vi "FetchVal34980a.vi"(0 "IP Address":string="localhost", 5 "TCP port":u16=5025 min=1025 step=1, 7 "Circuit ID":i32=1016 format="%_4g", 11 "error in (no error)":errorcluster) -> (4 "Value":dbl format="%#_10e", 15 "Error out":errorcluster)   [LabVIEW 2009]
doc: "Reads a value from the 34980. \nAssumes that you have scanned the 34980 to store the values."
panel:
  # "This assumes you have already scanned the 34980"
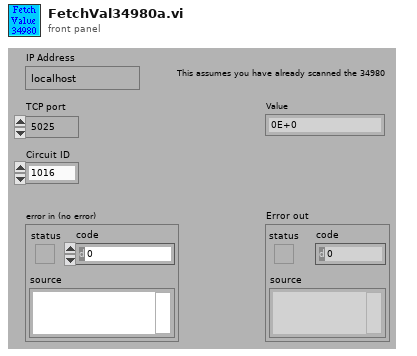
[diagram p1: front panel]
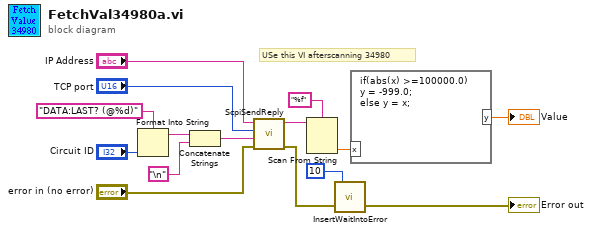
[diagram p0: block diagram]
diagram:
  # "USe this VI afterscanning 34980"
  n1 = Format Into String(format string="DATA:LAST? (@%d)", "Circuit ID") -> (resulting string=w10:string)  [unwired: 2 in, 1 out]
  n2 = Concatenate Strings(w10, "\n") -> (w8:string)
  n3 = call "ScpiSendReply.vi"("error in (no error)"="error in (no error)", "Command"=w8, "TCP port"="TCP port", "IP Address"="IP Address") -> ("Error out"=w7:errorcluster, "Reply"=w14:string)  [unwired: 5 in]
  n4 = Scan From String(format string="%f", input string=w14) -> (output 1=w4:dbl)  [unwired: 3 in, 3 out]
  n5 = call "InsertWaitIntoError.vi"("error in (no error)"=w7, "Wait (msecs)"=10) -> ("error out"=→"Error out":errorcluster)  [unwired: 1 in]
  n6 = formula code="if(abs(x) >=100000.0)\ny = -999.0;\nelse y = x;"("x"=w4) -> ("y"=→"Value":dbl)
